vi "GSI-HVSwitch2.trend data.vi"(0 "i ref in":refnum<vi>, 1 "ActVoltage":dbl, 3 "ms timeout (10000)":i32=10000, 5 "error in (no error)":errorcluster, 7 "ActTempAmp":dbl, 9 "ActTempPS1":dbl, 11 "ActTempPS2":dbl) -> (14 "i ref out":refnum<vi>, 17 "timed out":bool, 19 "error out":errorcluster)   [LabVIEW 2014, in "GSI-HVSwitch2.lvlib"]
doc: "Checks, if data has changed, writes it to the attribute data and publishes it via DIM."
uses:
  GSI-HVSwitch2.lvlib
  CSlibraries/UtilityLib/UtilityLib.valueStatus.ctl
  CSCore/CSApplicationBaseClasses/PSChannelBase/PSChannelBase.directionType.ctl
  CSCore/CSApplicationBaseClasses/PSChannelBase/PSChannelBase.serviceType.ctl
  CSCore/CSApplicationBaseClasses/PSChannelBase/PSChannelBase.statusType.ctl
  CSlibraries-extern/DimLVEvent/LVDimInterface/LVDimInterface.lvlib
  CSCore/CSApplicationBaseClasses/PSChannelBase/PSChannelBase.lvlib
  CSlibraries/UtilityLib/UtilityLib.lvlib
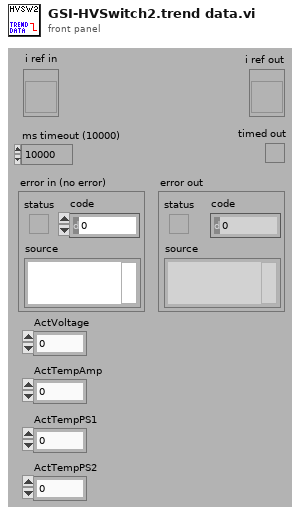
[diagram p1: front panel]
types:
  T1 = typedef "PSChannelBase.lvlib/PSChannelBase.directionType.ctl" = enum16{"unknown", "update actual value", "update nominal value", "update both"}
  T2 = typedef "UtilityLib.lvlib/UtilityLib.valueStatus.ctl" = enum16{"no info available", "stand by/off", "on", "warning", "alarm/malfunction", "not implemented", "user action required", "important information", "system default", "control default", "indicator default", "button default"}
  T3 = typedef "PSChannelBase.lvlib/PSChannelBase.serviceType.ctl" = enum16{"onOff", "voltage", "current", "tripCurrent", "rampUpSpeed", "rampDownSpeed", "status"}
  T4 = typedef "GSI-HVSwitch2.lvlib/GSI-HVSwitch2.i attribute.ctl" = cluster{"SDEX VISA Cluster":T5, "SetVoltage SW0":dbl, "SetVoltage SW1":dbl, "ActTempAmp":dbl, "ActTempPS1":dbl, "ActTempPS2":dbl, "mode":T8, "interfaceInitialized":bool, "serviceIDs":cluster{"nomVoltage0ID":i32, "nomVoltage1ID":i32, "actTempAmpID":i32, "actTempPS1ID":i32, "actTempPS2ID":i32, "modeID":i32}, "usedChannels":i32}
  T5 = typedef "SDEXDriver.lvlib/SDEX.VISA Control.ctl" = cluster{"VISA resource name":refnum<visa-resource-name>, "HEX address":u16, "VISA Timeout Value (1000 ms)":u32, "Lock Timeout (1000 ms)":u32, "semaphore":T6, "Baud rate":u32, "revision":T7, "deviceInfo":string}
  T6 = typedef "Semaphore RefNum" = refnum<k1>
  T7 = typedef "SDEXDriver.lvlib/SDEX.revisionType.ctl" = enum16{"unknown", "hvamp3", "hvswi1", "htrp0", "WDG0"}
  T8 = typedef "GSI-HVSwitch2.lvlib/GSI-HVSwitch2.mode.ctl" = enum16{"unknown", "switch", "stepper"}
  T9 = typedef "PSChannelBase.lvlib/PSChannelBase.i attribute.ctl" = cluster{"defaultChannelIndex":i32, "nofChannels":i32, "defaultChannelIndexID":i32, "nofChannelsID":i32, "actValues":T10, "nomValues":T10, "logicalName":string[], "physicalName":string[], "logicalNameID":i32, "physicalNameID":i32}
  T10 = typedef "PSChannelBase.lvlib/PSChannelBase.parameters.ctl" = cluster{"onOff":bool[], "voltage":dbl[], "current":dbl[], "tripCurrent":dbl[], "rampUpSpeed":dbl[], "rampDownSpeed":dbl[], "status":i32[], "serviceIDs":cluster{"onOfflID":i32, "voltageID":i32, "currentID":i32, "tripCurrentID":i32, "rampUpSpeedID":i32, "rampDownSpeedID":i32, "statusID":i32}}
  T11 = typedef "PSChannelBase.lvlib/PSChannelBase.statusType.ctl" = i32
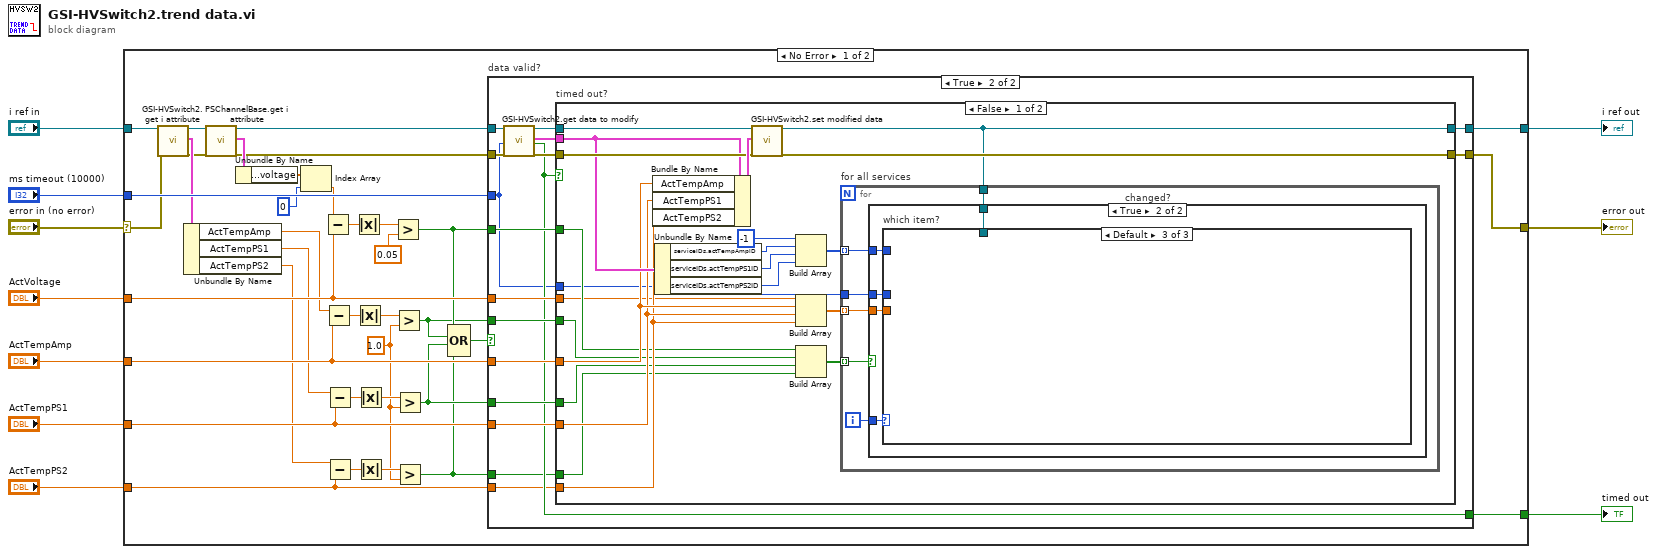
[diagram p0: block diagram]
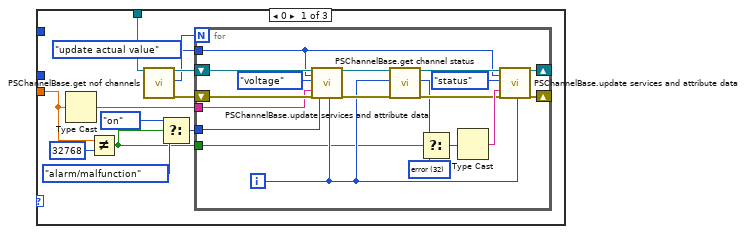
[diagram p4: hidden frame]
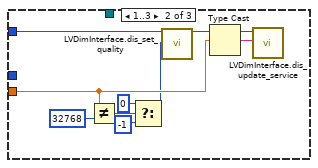
[diagram p5: hidden frame]
diagram:
  n1 = case shown="No Error" "error in (no error)" {
    selector: "error in (no error)" -> [w19 w142]
    tunnel: [w47 w142] -> w10
    tunnel: [w46 w143] -> w9
    tunnel: "ms timeout (10000)" -> [w45 _]
    tunnel: "i ref in" -> [w44 w143]
    tunnel: "ActVoltage" -> [w42 _]
    tunnel: "ActTempAmp" -> [w35 _]
    tunnel: "ActTempPS1" -> [w30 _]
    tunnel: [w26 _] -> w3
    tunnel: "ActTempPS2" -> [w21 _]
    frame No Error {
      w23 = 1.0 ("y")
      n2 = call "GSI-HVSwitch2.get i attribute.vi"("i ref in"=w44, "error in (no error)"=w19) -> ("i ref out"=w18:refnum<vi>, "i attribute"=w43:T4, "error out"=w17:errorcluster)  [unwired: 15 in]
      n3 = Unbundle By Name(w43) -> ("ActTempAmp"=w36:dbl, "ActTempPS1"=w32:dbl, "ActTempPS2"=w22:dbl)
      n4 = call "PSChannelBase.get i attribute.vi"("i ref in"=w18, "error in (no error)"=w17) -> ("i ref out"=w12:refnum<vi>, "i attribute"=w16:T9, "error out"=w11:errorcluster)  [unwired: 15 in]
      n5 = Unbundle By Name(w16) -> ("actValues.voltage"=w15:dbl[])
      n6 = Index Array(array=w15, index=0) -> (element=w14:dbl)
      n7 = Subtract(x=w14, y=w42) -> (x-y=w41:dbl)
      n8 = Subtract(x=w36, y=w35) -> (x-y=w37:dbl)
      n9 = Subtract(x=w32, y=w30) -> (x-y=w34:dbl)
      n10 = Subtract(x=w22, y=w21) -> (x-y=w24:dbl)
      n11 = Absolute Value(x=w41) -> (abs(x)=w40:dbl)
      n12 = Absolute Value(x=w37) -> (abs(x)=w38:dbl)
      n13 = Absolute Value(x=w34) -> (abs(x)=w33:dbl)
      n14 = Absolute Value(x=w24) -> (abs(x)=w25:dbl)
      n15 = Greater?(x=w40, y=0.05) -> (0:w29:bool)
      n16 = Greater?(x=w38, y=w23) -> (0:w28:bool)
      n17 = Greater?(x=w33, y=w23) -> (0:w27:bool)
      n18 = Greater?(x=w25, y=w23) -> (0:w20:bool)
      n19 = Compound Arithmetic op=OR(w29, w28, w27, w20) -> (w31:bool)
      n20 = case "data valid?" shown="True" w31 {
        tunnel: [w48 w66] -> w47
        tunnel: [w49 w65] -> w46
        tunnel: w45 -> [_ w50]
        tunnel: w42 -> [_ w61]
        tunnel: w35 -> [_ w60]
        tunnel: w12 -> [w49 w59]
        tunnel: w11 -> [w48 w58]
        tunnel: w30 -> [_ w57]
        tunnel: w29 -> [_ w56]
        tunnel: w28 -> [_ w55]
        tunnel: w27 -> [_ w54]
        tunnel: [_ w53] -> w26
        tunnel: w21 -> [_ w52]
        tunnel: w20 -> [_ w51]
        frame False {
        }
        frame True {
          n21 = call "GSI-HVSwitch2.get data to modify.vi"("i ref in"=w59, "ms timeout (10000)"=w50, "error in (no error)"=w58) -> ("i ref out"=w63:refnum<vi>, "i attribute"=w62:T4, "timed out"=w53:bool, "error out"=w64:errorcluster)  [unwired: 13 in]
          n22 = case "timed out?" shown="False" w53 {
            tunnel: [w84 w140] -> w66
            tunnel: [w68 w141] -> w65
            tunnel: w61 -> [w70 _]
            tunnel: w60 -> [w80 _]
            tunnel: w64 -> [w86 w140]
            tunnel: w63 -> [w87 w141]
            tunnel: w62 -> [w85 _]
            tunnel: w57 -> [w79 _]
            tunnel: w56 -> [w77 _]
            tunnel: w55 -> [w76 _]
            tunnel: w54 -> [w75 _]
            tunnel: w52 -> [w78 _]
            tunnel: w51 -> [w74 _]
            tunnel: w50 -> [w67 _]
            frame False {
              n23 = Bundle By Name(cluster=w85, "ActTempAmp"=w80, "ActTempPS1"=w79, "ActTempPS2"=w78) -> (w88:T4)
              n24 = Unbundle By Name(w85) -> ("serviceIDs.actTempAmpID"=w83:i32, "serviceIDs.actTempPS1ID"=w82:i32, "serviceIDs.actTempPS2ID"=w81:i32)
              n25 = call "GSI-HVSwitch2.set modified data.vi"("i ref in"=w87, "i attribute"=w88, "error in (no error)"=w86) -> ("i ref out"=w68:refnum<vi>, "error out"=w84:errorcluster)  [unwired: 15 in]
              n26 = Build Array(-1 ("element"), w83, w82, w81) -> (w73:i32[])
              n27 = Build Array(w70, w80, w79, w78) -> (w72:dbl[])
              n28 = Build Array(w77, w76, w75, w74) -> (w71:bool[])
              n29 = for "for all services" {
                tunnel: w73 -> [w92] mode=indexing
                tunnel: w72 -> [w93] mode=indexing
                tunnel: w71 -> [w94] mode=indexing
                tunnel: w68 -> [w90]
                tunnel: w67 -> [w89]
                i -> [w91]
                n30 = case "changed?" shown="True" w94 {
                  tunnel: w93 -> [_ w98]
                  tunnel: w92 -> [_ w99]
                  tunnel: w91 -> [_ w97]
                  tunnel: w90 -> [_ w96]
                  tunnel: w89 -> [_ w95]
                  frame False {
                  }
                  frame True {
                    n31 = case "which item?" shown="Default" w97 {
                      tunnel: w99 -> [_ w134 _]
                      tunnel: w98 -> [w109 w132 _]
                      tunnel: w96 -> [w111 _ _]
                      tunnel: w95 -> [_ _ _]
                      frame 0 {
                        n32 = Type Cast(x=w109) -> (*(type *) &x=w104:string)  [unwired: 1 in]
                        n33 = Not Equal?(x=w109, y=u16 32768) -> (x != y?=w101:bool)
                        n34 = call "PSChannelBase.get nof channels.vi"("i ref in"=w111) -> ("i ref out"=w106:refnum<vi>, "NofChannels"=w102:i32, "error out"=w105:errorcluster)  [unwired: 16 in]
                        n35 = Select(t=UtilityLib.valueStatus."on" ("quality"), s=w101, f=UtilityLib.valueStatus."alarm/malfunction") -> (s? t:f=w103:T2)
                        n36 = for {
                          N: w102 -> [_]
                          tunnel: w104 -> [w128]
                          tunnel: w103 -> [w127]
                          shift-right: [w117] -> _
                          shift-left: w106 -> [w130]
                          shift-right: [w116] -> _
                          shift-left: w105 -> [w129]
                          tunnel: w101 -> [w114]
                          tunnel: PSChannelBase.directionType."update actual value" ("direction") -> [w112]
                          i -> [w115]
                          w126 = T11 32 items=["onOff"=1, "inRange"=2, "rampingUp"=4, "rampingDown"=8, "tripped"=16, "error"=32] ("service")
                          n37 = call "PSChannelBase.update services and attribute data.vi"("i ref in"=w130, "direction"=w112, "service"=PSChannelBase.serviceType."voltage", "value"=w128, "error in (no error)"=w129, "quality"=w127, "channelNumber"=w115) -> ("i ref out"=w118:refnum<vi>, "error out"=w119:errorcluster)  [unwired: 10 in, 1 out]
                          n38 = call "PSChannelBase.get channel status.vi"("i ref in"=w118, "channelIndex"=w115, "error in (no error)"=w119) -> ("i ref out"=w122:refnum<vi>, "status"=w120:i32, "error out"=w121:errorcluster)  [unwired: 14 in]
                          n39 = Select(t=w120, s=w114, f=w126) -> (s? t:f=w125:T11)
                          n40 = Type Cast(x=w125) -> (*(type *) &x=w123:string)  [unwired: 1 in]
                          n41 = call "PSChannelBase.update services and attribute data.vi"("i ref in"=w122, "direction"=w112, "service"=PSChannelBase.serviceType."status", "value"=w123, "error in (no error)"=w121, "channelNumber"=w115) -> ("i ref out"=w117:refnum<vi>, "error out"=w116:errorcluster)  [unwired: 11 in, 1 out]
                        }
                      }
                      frame 1..3 {
                        n42 = Not Equal?(x=w132, y=u16 32768) -> (x != y?=w137:bool)
                        n43 = Select(t=0, s=w137, f=-1) -> (s? t:f=w131:i32)
                        n44 = call "LVDimInterface.dis_set_quality.vi"("my_serviceID"=w134, "quality"=w131) -> ("my_serviceID (out)"=w133:i32)  [unwired: 16 in, 1 out]
                        n45 = Type Cast(x=w132) -> (*(type *) &x=w139:string)  [unwired: 1 in]
                        n46 = call "LVDimInterface.dis_update_service.vi"("my_serviceID"=w133, "data"=w139) -> ()  [unwired: 15 in, 3 out]
                      }
                      frame Default {
                      }
                    }
                  }
                }
              }
            }
            frame True {
            }
          }
        }
      }
    }
    frame Error {
    }
  }
  "error out" <- w10
  "i ref out" <- w9
  "timed out" <- w3
